vi "FixDataRootInXML.vi"(9 "pathPlaceholderString":string, 10 "replacementPath":string, 11 "XMLstringIn":string) -> (3 "XMLstringOut":string)   [LabVIEW 2022 SP3]
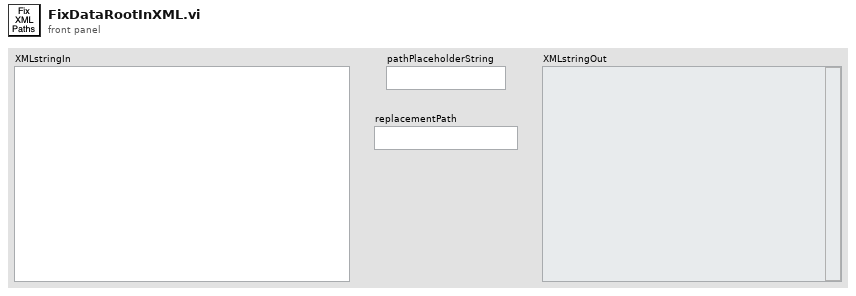
[diagram p1: front panel]
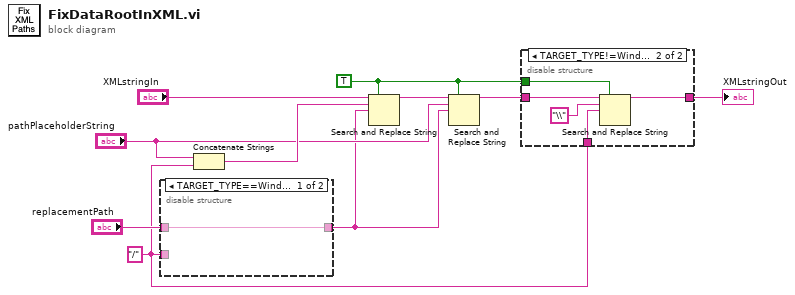
[diagram p0: block diagram]
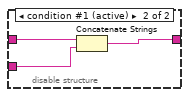
[diagram p3: hidden frame]
diagram:
  w1 = "/" ("string")
  w2 = TRUE ("replace all? (F)")
  n1 = disable-structure shown="TARGET_TYPE==Windows, Default" {
    disable-tunnel: [w11 w13] -> w5
    disable-tunnel: "replacementPath" -> [w11 w14]
    disable-tunnel: w1 -> [_ w12]
    frame condition #0 {
    }
    frame condition #1 (active) {
      n2 = Concatenate Strings(w14, w12) -> (w13:string)
    }
  }
  n3 = Concatenate Strings("pathPlaceholderString", w1) -> (w8:string)
  n4 = Search and Replace String(replace all?=w2, input string="XMLstringIn", search string=w8, replace string=w5) -> (result string=w7:string)  [unwired: 4 in, 3 out]
  n5 = Search and Replace String(replace all?=w2, input string=w7, search string="pathPlaceholderString", replace string=w5) -> (result string=w3:string)  [unwired: 4 in, 3 out]
  n6 = disable-structure shown="TARGET_TYPE!=Windows" {
    disable-tunnel: [w15 w18] -> w4
    disable-tunnel: w3 -> [w15 w19]
    disable-tunnel: w2 -> [_ w17]
    disable-tunnel: w1 -> [_ w16]
    frame condition #0 {
    }
    frame condition #1 (active) {
      n7 = Search and Replace String(replace all?=w17, input string=w19, search string="\\", replace string=w16) -> (result string=w18:string)  [unwired: 4 in, 3 out]
    }
  }
  "XMLstringOut" <- w4
